vi "BuildTitleString.vi"(0 "tagged text":string, 1 "ROS":T1={"topic port"=0, "Node"="", "topic"="", "type"="", "node port"=0, "error "={"status"=FALSE, "code"=0, "source"=""}, "Direction"=enum."Node", "Update (ms)"=1, "FIFO size"=0}) -> (2 "String":string)   [LabVIEW 2016]
doc: "Builds title string for website logs"
uses:
  _ROSControl.ctl
  _ROSDirection.ctl
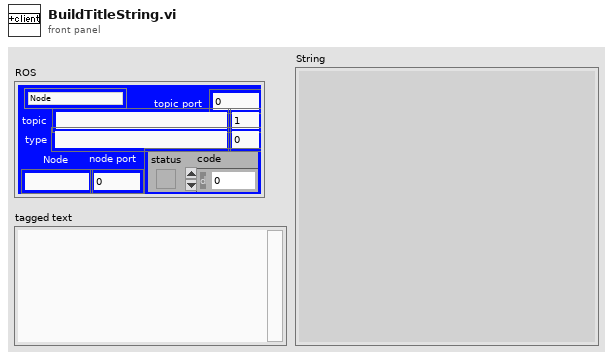
[diagram p1: front panel]
types:
  T1 = typedef "_ROSControl.ctl" = cluster{"topic port":u16, "Node":string, "topic":string, "type":string, "node port":u16, "error ":errorcluster, "Direction":T2, "Update (ms)":u16, "FIFO size":u16}
  T2 = typedef "_ROSDirection.ctl" = enum16{"Node", "Publisher", "Subscriber", "ServiceClient", "ServiceProvider"}
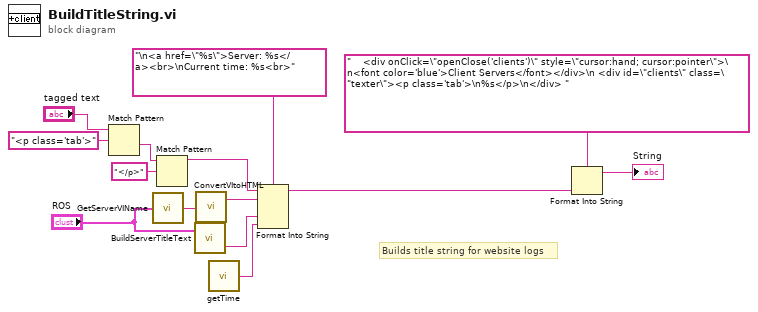
[diagram p0: block diagram]
diagram:
  # "Builds title string for website logs"
  n1 = Match Pattern(string="tagged text", regular expression="<p class='tab'>") -> (after substring=w4:string)  [unwired: 1 in, 3 out]
  n2 = call "GetServerVIName.vi"("ROS"="ROS") -> ("vi name"=w2:string)
  n3 = Match Pattern(string=w4, regular expression="</p>") -> (before substring=w3:string)  [unwired: 1 in, 3 out]
  n4 = call "BuildServerTitleText.vi"("ROS"="ROS") -> ("text"=w14:string)  [unwired: 1 in, 1 out]
  n5 = call "ConvertVItoHTML.vi"("vi name"=w2) -> ("Htm log name"=w1:string)  [unwired: 1 out]
  n6 = call "getTime.vi"() -> ("Current Time"=w10:string)  [unwired: 1 in]
  n7 = Format Into String(format string="\n<a href=\"%s\">Server: %s</a><br>\nCurrent time: %s<br>" ("regular expression"), initial string=w3, w1, w14, w10) -> (resulting string=w11:string)  [unwired: 1 in, 1 out]
  n8 = Format Into String(format string="    <div onClick=\"openClose('clients')\" style=\"cursor:hand; cursor:pointer\">\n<font color='blue'>Client Servers</font></div>\n <div id=\"clients\" class=\"texter\"><p class='tab'>\n%s</p>\n</div> " ("regular expression"), w11) -> (resulting string=→"String":string)  [unwired: 2 in, 1 out]
